vi "LabView_FC.vi"() -> ()   [LabVIEW 2013]
panel:
  in  "Range (1,2,3,4) AutoRange - 255":dbl=10.0 caption="Range" min=0.0 max=255.0 step=1.0 format="%#_3f"
  in  "Sampling Time (Sec)":dbl=10.0 min=0.1 max=10.0 step=0.1 format="%#_2g"
  out "Frequncy Read (MHz)":dbl format="%#_14g"
  in  "MCL_FreqCounter._USB_FreqCounter":refnum<k7> caption="UFC-6000"
  in  "stop":bool
  # "____________________________________________________________________________________________________"
  # "-  This is an example Of Mini-Circuits UFC-6000 Frequency Counter.\n-  The example use an acticeX , so before using this example make sure to install MCL_FreqCounter.dll \n-  To close the application , use the Stop Button . other wise disconnect and reconnect the Power meter to the USB port"
  # "Mini Circuits  UFC-6000 Frequency Counter"
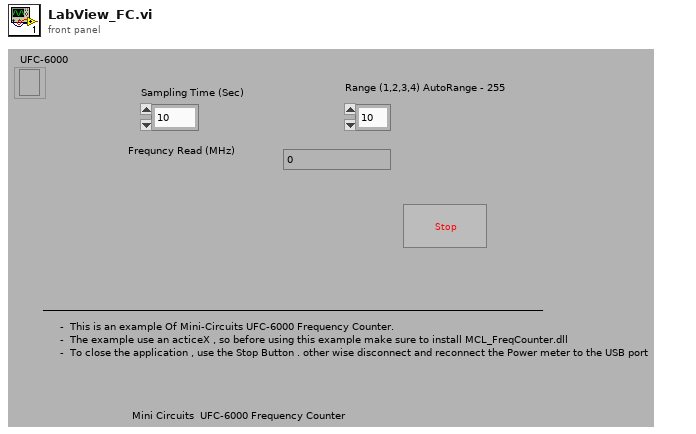
[diagram p1: front panel]
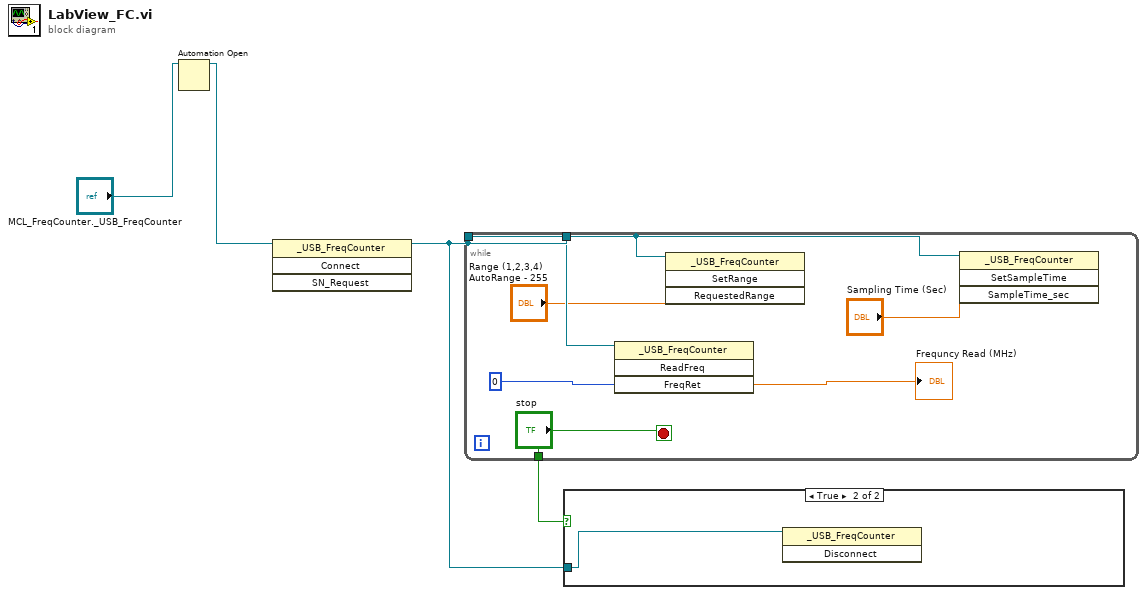
[diagram p0: block diagram]
diagram:
  n1 = Automation Open(Automation Refnum="MCL_FreqCounter._USB_FreqCounter") -> (Automation Refnum=w1:refnum<k7>)  [unwired: 3 in, 1 out]
  n2 = invoke class="_USB_FreqCounter" method="Connect"(reference=w1) -> (reference out=w2:refnum<k7>)  [unwired: 3 in, 3 out]
  n3 = while {
    tunnel: ["stop"] -> w4
    tunnel: w2 -> [w10]
    tunnel: w2 -> [w7]
    stop <- "stop" stop-if-true
    n4 = invoke class="_USB_FreqCounter" method="ReadFreq"(reference=w10, "FreqRet"=0) -> ("FreqRet"=→"Frequncy Read (MHz)":dbl)  [unwired: 2 in, 3 out]
    n5 = invoke class="_USB_FreqCounter" method="SetRange"(reference=w7, "RequestedRange"="Range (1,2,3,4) AutoRange - 255") -> ()  [unwired: 2 in, 4 out]
    n6 = invoke class="_USB_FreqCounter" method="SetSampleTime"(reference=w7, "SampleTime_sec"="Sampling Time (Sec)") -> ()  [unwired: 2 in, 4 out]
  }
  n7 = case shown="True" w4 {
    tunnel: w2 -> [_ w12]
    frame False {
    }
    frame True {
      n8 = invoke class="_USB_FreqCounter" method="Disconnect"(reference=w12) -> ()  [unwired: 2 in, 3 out]
    }
  }
